vi "RANGE Cubic Foot Per Hour.vi"(8 "Error In":errorcluster, 9 "Ft³/HR Factor":dbl, 10 "Reference Voltage":dbl, 11 "DAQ Output (Voltage)":dbl) -> (0 "Error Out":errorcluster, 3 "Ft³/HR":dbl)   [LabVIEW 2016]
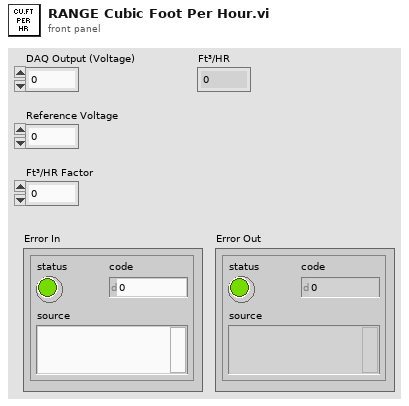
[diagram p1: front panel]
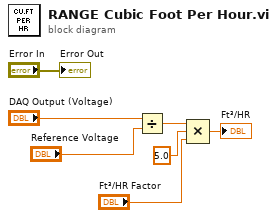
[diagram p0: block diagram]
diagram:
  n1 = Divide(x="DAQ Output (Voltage)", y="Reference Voltage") -> (x/y=w5:dbl)
  n2 = Compound Arithmetic op=MULTIPLY(w5, 5.0, "Ft³/HR Factor") -> (→"Ft³/HR":dbl)
  "Error Out" <- "Error In"
